vi "GetChannelMask.vi"(1 "ChainNumber":u8) -> (0 "ChainMask":u8)   [LabVIEW 2023, in "ArduinoSerialBling.lvlib"]
uses:
  ArduinoSerialBling.lvlib
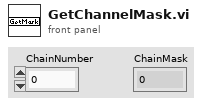
[diagram p1: front panel]
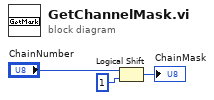
[diagram p0: block diagram]
diagram:
  n1 = Logical Shift(y="ChainNumber", x=u8 1) -> (x << y=→"ChainMask":u8)
